vi "传感器读取.vi"() -> ()   [LabVIEW 2020]
uses:
  <vilib>/Instr/_visa.llb/VISA Configure Serial Port (Instr).vi
  Global_Variable/Global.vi
panel:
  out "source":string caption="源"
  out "error out":cluster{"status":bool, "code":i32} caption="错误输出"
  in  "error in (no error)":errorcluster caption="错误输入（无错误）"
  out "数值 4":dbl format="%#_13g"
  out "数值 3":dbl format="%#_13g"
  out "数值 2":dbl format="%#_13g"
  out "数值 1":dbl format="%#_13g"
  in  "停止":bool
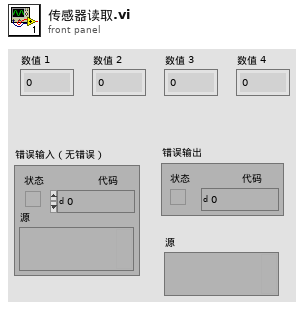
[diagram p1: front panel]
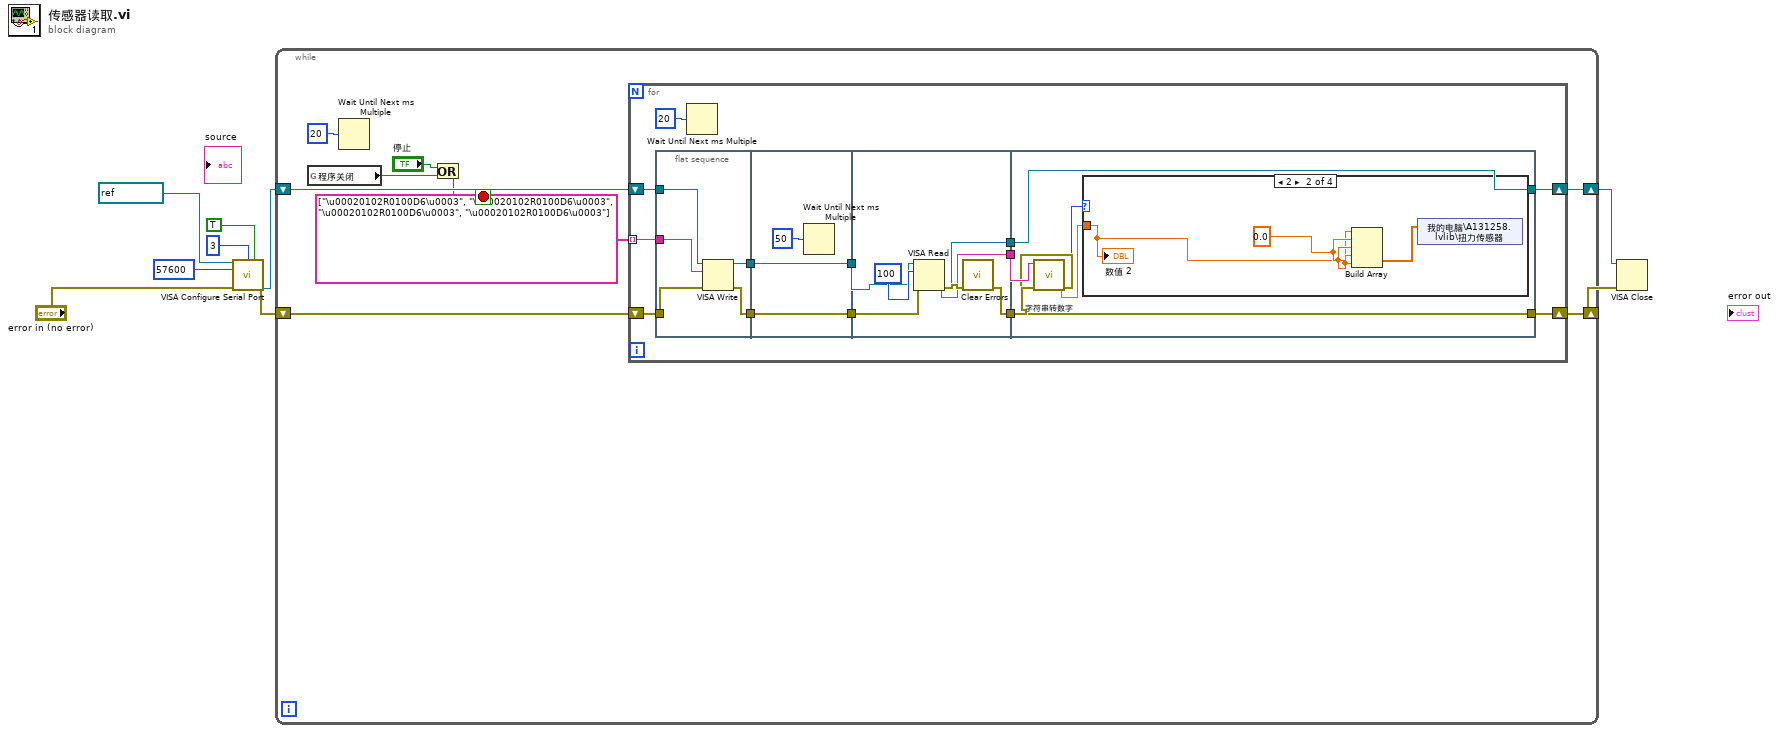
[diagram p0: block diagram]
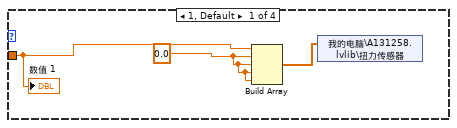
[diagram p2: hidden frame]
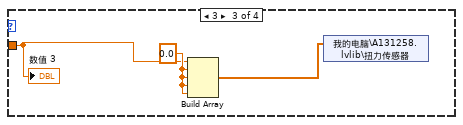
[diagram p3: hidden frame]
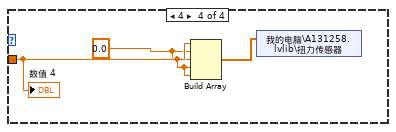
[diagram p4: hidden frame]
diagram:
  n1 = call-poly "VISA Configure Serial Port"("VISA resource name"=refnum<visa-resource-name> "COM3", "termination char\n(0xA = '\\n' = LF)"=u8 3 ("termination char\n(0xA = '\\n' = LF)"), "Enable Termination\nChar (T)"=TRUE ("Enable Termination\nChar (T)"), "baud rate (9600)"=u32 57600, "error in (no error)"="error in (no error)") -> ("VISA resource name out"=w4:refnum<visa-resource-name>, "error out"=w2:errorcluster)  [unwired: 9 in]
  n2 = while {
    shift-right: [w16] -> w9
    shift-left: w4 -> [w17]
    shift-right: [w13] -> w7
    shift-left: w2 -> [w14]
    stop <- w11 stop-if-true
    n3 = global read "Global.vi" "程序关闭"() -> (w10:bool)
    n4 = Wait Until Next ms Multiple(millisecond multiple=u32 20 ("毫秒倍数")) -> ()  [unwired: 1 out]
    n5 = Or(x="停止", y=w10) -> (x .or. y?=w11:bool)
    n6 = for {
      tunnel: string[] ["\u00020102R0100D6\u0003", "\u00020102R0100D6\u0003", "\u00020102R0100D6\u0003", "\u00020102R0100D6\u0003"] ("写入缓冲区") -> [w30] mode=indexing
      shift-right: [w21] -> w16
      shift-left: w17 -> [w31]
      shift-right: [w19] -> w13
      shift-left: w14 -> [w29]
      n7 = flat-sequence {
        tunnel: w31 -> [w36]
        tunnel: w30 -> [w34]
        tunnel: w29 -> [w33]
        tunnel: [w35] -> w28
        tunnel: [w32] -> w27
        tunnel: w28 -> [w39]
        tunnel: w27 -> [w38]
        tunnel: [w39] -> w26
        tunnel: [w38] -> w25
        tunnel: w26 -> [w44]
        tunnel: w25 -> [w46]
        tunnel: [w40] -> w24
        tunnel: [w42] -> w23
        tunnel: [w41] -> w22
        tunnel: [w52] -> w21
        tunnel: [w49] -> w19
        tunnel: w24 -> [w50]
        tunnel: w23 -> [w51]
        tunnel: w22 -> [w52]
        frame #0 {
          n8 = VISA Write(VISA resource name=w36, write buffer=w34, error in (no error)=w33) -> (VISA resource name out=w35:refnum<visa-resource-name>, error out=w32:errorcluster)  [unwired: 1 out]
        }
        frame #1 {
          n9 = Wait Until Next ms Multiple(millisecond multiple=u32 50 ("毫秒倍数")) -> ()  [unwired: 1 out]
        }
        frame #2 {
          n10 = VISA Read(VISA resource name=w44, byte count=u32 100 ("字节总数"), error in (no error)=w46) -> (VISA resource name out=w41:refnum<visa-resource-name>, read buffer=w42:string, error out=w43:errorcluster)  [unwired: 1 out]
          n11 = call <vilib>:"Clear Errors.vi"("error in (no error)"=w43) -> ("error out"=w40:errorcluster)  [unwired: 5 in, 1 out]
        }
        frame #3 {
          n12 = call "字符串转数字.vi"("error in (no error)"=w50, "字符串"=w51) -> ("error out"=w49:errorcluster, "数值"=w47:dbl, "ID"=w48:i32)  [unwired: 7 in]
          n13 = case shown="2" w48 {
            tunnel: w47 -> [w53 w56 w59 w63]
            frame 1, Default {
              w54 = 0.0 ("元素")
              n14 = Build Array(w53, w54, w54, w54, w54) -> (w55:dbl[])
              n15 = shared-variable "我的电脑\\A131258.lvlib\\扭力传感器"(w55) -> ()  [unwired: 1 in, 1 out]
              "数值 1" <- w53
            }
            frame 2 {
              w57 = 0.0 ("元素")
              n16 = Build Array(w56, w57, w57, w57, w57) -> (w58:dbl[])
              n17 = shared-variable "我的电脑\\A131258.lvlib\\扭力传感器"(w58) -> ()  [unwired: 1 in, 1 out]
              "数值 2" <- w56
            }
            frame 3 {
              w60 = 0.0 ("元素")
              n18 = Build Array(w59, w60, w60, w60, w60) -> (w61:dbl[])
              n19 = shared-variable "我的电脑\\A131258.lvlib\\扭力传感器"(w61) -> ()  [unwired: 1 in, 1 out]
              "数值 3" <- w59
            }
            frame 4 {
              w62 = 0.0 ("元素")
              n20 = Build Array(w63, w62, w62, w62, w62) -> (w64:dbl[])
              n21 = shared-variable "我的电脑\\A131258.lvlib\\扭力传感器"(w64) -> ()  [unwired: 1 in, 1 out]
              "数值 4" <- w63
            }
          }
        }
      }
      n22 = Wait Until Next ms Multiple(millisecond multiple=u32 20 ("毫秒倍数")) -> ()  [unwired: 1 out]
    }
  }
  n23 = VISA Close(VISA resource name=w9, error in (no error)=w7) -> ()  [unwired: 1 out]
